vi "Write States.vi"(8 "error in (no error)":errorcluster, 10 "States":enum16{"PassObserver", "Exit"}(ring), 11 "PassObserverTactic in":refnum<class "PassObserverTactic.lvclass">) -> (0 "error out":errorcluster, 3 "PassObserverTactic out":refnum<class "PassObserverTactic.lvclass">)   [LabVIEW 2018, in "PassObserverTactic.lvclass"]
uses:
  PassObserverTactic.lvclass
  PassObserverTactic.lvclass/PassObserverTactic.ctl
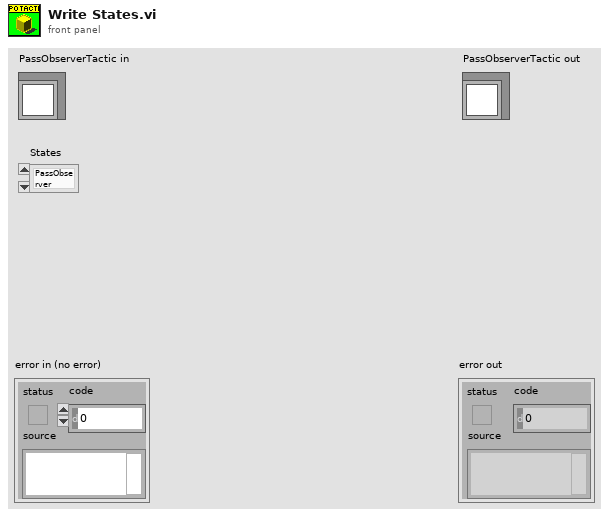
[diagram p1: front panel]
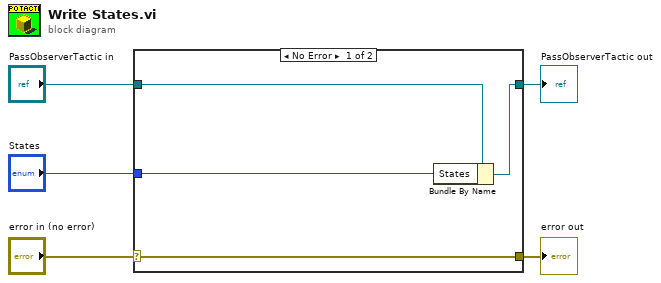
[diagram p0: block diagram]
diagram:
  n1 = case shown="No Error" "error in (no error)" {
    selector: "error in (no error)" -> [w9 w10]
    tunnel: [w9 w10] -> w4
    tunnel: [w7 w11] -> w2
    tunnel: "PassObserverTactic in" -> [w8 w11]
    tunnel: "States" -> [w6 _]
    frame No Error {
      n2 = Bundle By Name(cluster=w8, "States"=w6) -> (w7:refnum<class "PassObserverTactic.lvclass">)
    }
    frame Error {
    }
  }
  "error out" <- w4
  "PassObserverTactic out" <- w2
